vi "Receive message.vi"(8 "error in (no error)":errorcluster, 11 "Server in":refnum<class "TCP-Server.lvclass">) -> (0 "error out":errorcluster, 1 "isAcommand":bool, 2 "message":string, 3 "Server out":refnum<class "TCP-Server.lvclass">)   [LabVIEW 2018, in "TCP-Server.lvclass"]
uses:
  TCP-Server.lvclass
  TCP-Server.lvclass/TCP-Server.ctl
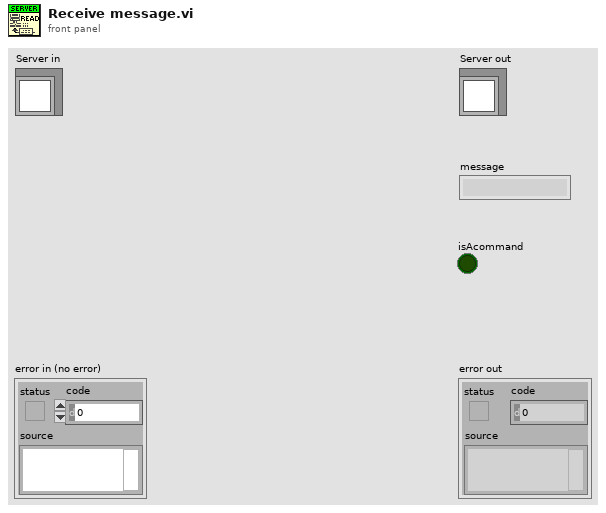
[diagram p1: front panel]
types:
  T1 = enum16{"Standard", "Buffered", "CRLF", "Immediate"}
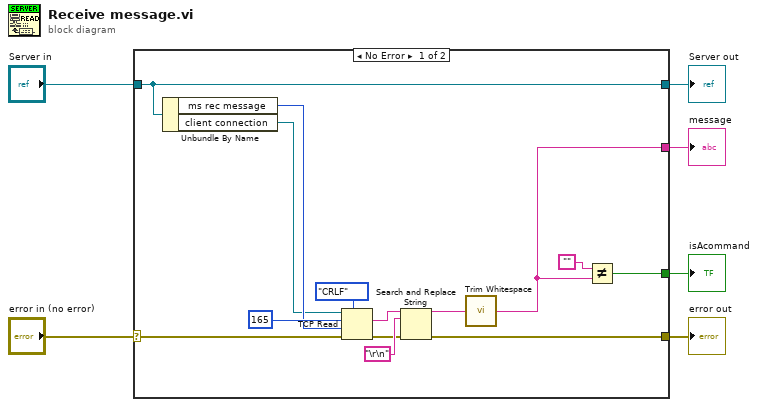
[diagram p0: block diagram]
diagram:
  n1 = case shown="No Error" "error in (no error)" {
    selector: "error in (no error)" -> [w13 w21]
    tunnel: [w12 w21] -> w5
    tunnel: [w20 w22] -> w3
    tunnel: "Server in" -> [w20 w22]
    tunnel: [w8 _] -> w2
    tunnel: [w9 _] -> w1
    frame No Error {
      n2 = Unbundle By Name(w20) -> ("ms rec message"=w11:i32, "client connection"=w10:refnum<k5>)
      n3 = TCP Read(connection ID=w10, bytes to read=165, error in (no error)=w13, 7:T1."CRLF" ("mode (standard)"), 9:w11) -> (data out=w15:string, error out=w14:errorcluster)  [unwired: 1 out]
      n4 = Search and Replace String(input string=w15, search string="\r\n", error in=w14) -> (result string=w16:string, error out=w12:errorcluster)  [unwired: 5 in, 2 out]
      n5 = call <vilib>:"Trim Whitespace.vi"("string"=w16) -> ("trimmed string"=w8:string)  [unwired: 1 in]
      n6 = Not Equal?(x="", y=w8) -> (x != y?=w9:bool)
    }
    frame Error {
    }
  }
  "error out" <- w5
  "Server out" <- w3
  "message" <- w2
  "isAcommand" <- w1
